vi "fw103_with_subvi_errorhandle.vi"(7 "SerialNumber":string="40154488", 8 "Set position\n(deg) (float)":dbl, 9 "Move (bool)":bool, 10 "Stop all (bool)":bool) -> (0 "Polling reference":refnum<k24>, 1 "Method reference":refnum<k24>, 3 "Current position (deg) (float)":i32)   [LabVIEW 2020]
uses:
  C:/Users/OPMuser/Documents/labview/fw103/Thorlabs.MotionControl.Benchtop.StepperMotorCLI.dll
  Thorlabs.MotionControl.Benchtop.StepperMotorCLI.dll
  <extravilib>/ChannelInstances/Tag-bool.lvlib
  <extravilib>/ChannelInstances/Stream-bool.lvlib
  <vilib>/ErrorRing/Error Ring.xnode
  <vilib>/Utility/error.llb/Error Cluster From Error Code.vi
  C:/Users/OPMuser/Documents/labview/fw103/Thorlabs.MotionControl.Controls.dll
  Thorlabs.MotionControl.Controls.dll
panel:
  in  "Set/Move":dbl
  # "Filter wheel control"
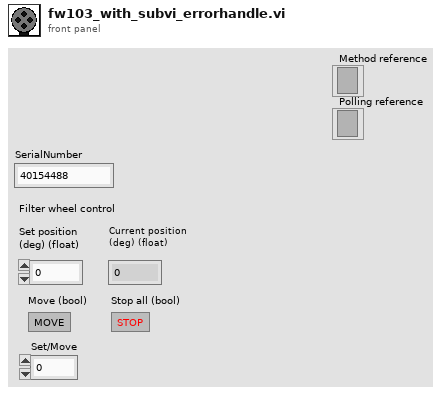
[diagram p1: front panel]
types:
  T1 = typedef "Tag-bool.lvlib/))Channel.ctl" = refnum<queue>
  T2 = typedef "Stream-bool.lvlib/)Channel.ctl" = refnum<queue>
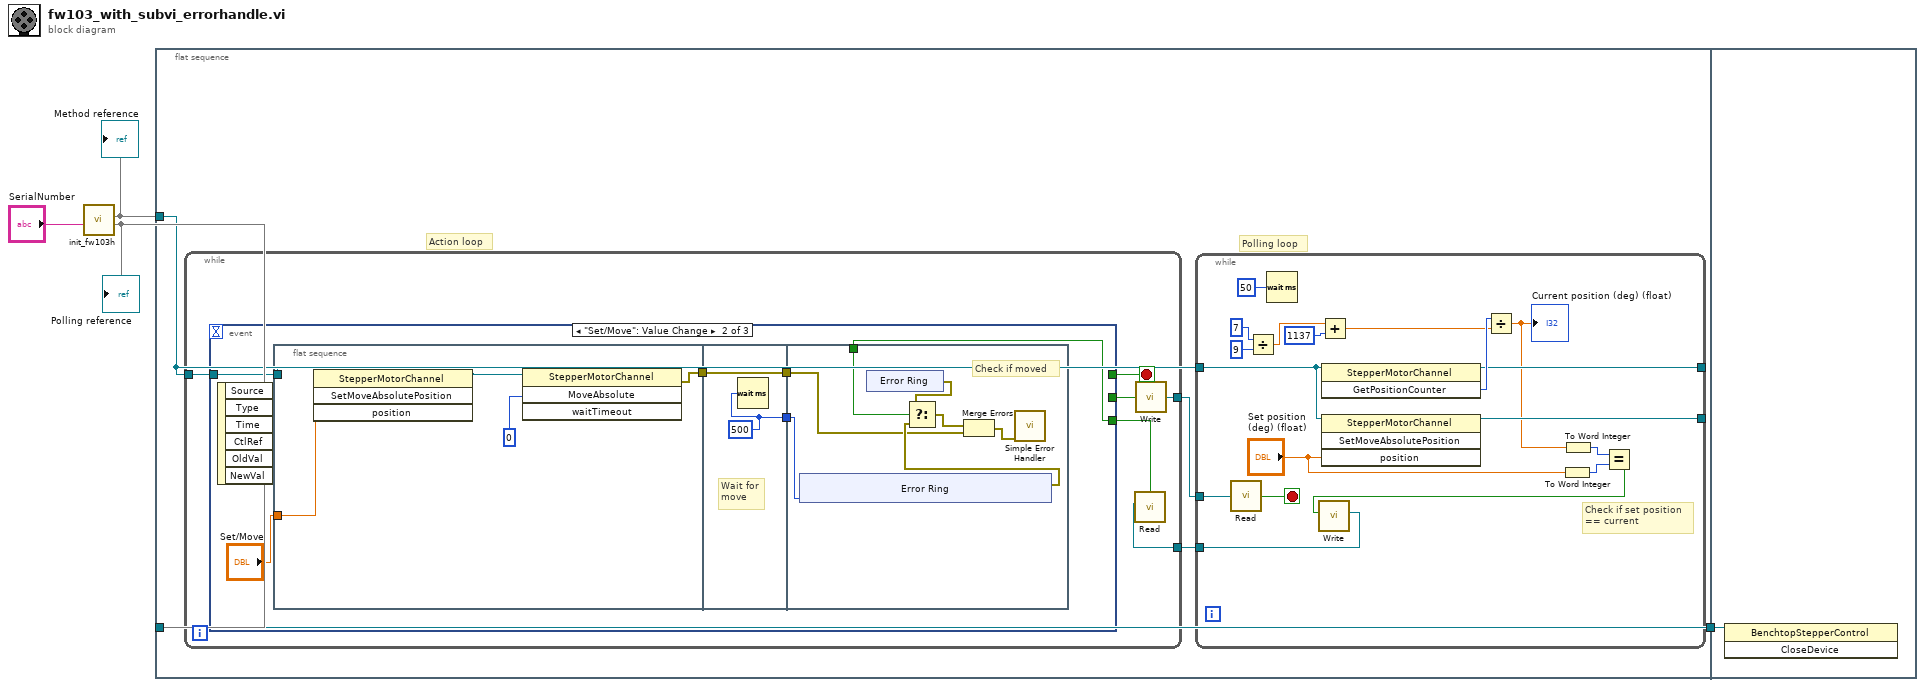
[diagram p0: block diagram]
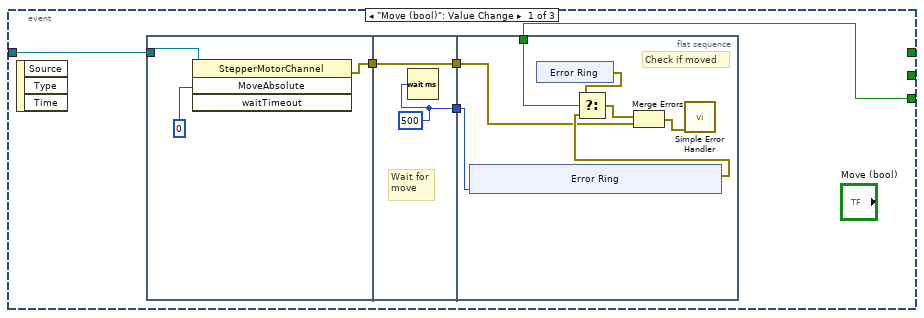
[diagram p2: hidden frame]
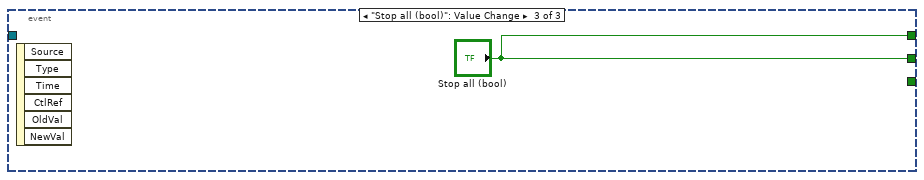
[diagram p3: hidden frame]
diagram:
  n1 = call "init_fw103h.vi"("SerialNumber"="SerialNumber") -> (1:w2, 2:w4)  [unwired: 8 in, 1 out]
  "Method reference" <- w4
  "Polling reference" <- w2
  n2 = flat-sequence {
    tunnel: w4 -> [w6]
    tunnel: [w8] -> w3
    tunnel: w2 -> [w8]
    tunnel: w3 -> [w87]
    frame #0 {
      # "Action loop"
      # "Polling loop"
      n3 = while {
        tunnel: [w12] -> w7
        tunnel: w6 -> [w11]
        tunnel: w5 -> [w9]
        stop <- w14 stop-if-true
        n4 = call <extravilib>:"Read.vi"("channel"=w9) -> ("element"=w10:bool)  [unwired: 6 in, 4 out]
        n5 = event shown="[1] \"Set/Move\": Value Change" {
          selector: _ -> [_ _ _]
          dyn-events: _ -> [_ _ _]
          timeout: _ -> [_ _ _]
          tunnel: [_ _ "Stop all (bool)"] -> w14
          tunnel: [_ _ "Stop all (bool)"] -> w13
          tunnel: w11 -> [w19 w42 _]
          tunnel: w10 -> [w17 w41 _]
          event "Move (bool)": Value Change {
            n6 = event-data() -> ()  [unwired: 1 in, 3 out]
            n7 = flat-sequence {
              tunnel: w19 -> [w21]
              tunnel: [w20] -> w15
              tunnel: [w24] -> w18
              tunnel: [w23] -> w16
              tunnel: w15 -> [w23]
              tunnel: w18 -> [w31]
              tunnel: w17 -> [w30]
              tunnel: w16 -> [w26]
              frame #0 {
                n8 = invoke class="StepperMotorChannel" method="MoveAbsolute"(reference=w21, "waitTimeout"=0) -> (error out=w20:errorcluster)  [unwired: 2 in, 3 out]
              }
              frame #1 {
                w24 = 500 ("waitTimeout")
                # "Wait for\nmove"
                n9 = Wait (ms)(milliseconds to wait=w24) -> ()  [unwired: 1 out]
              }
              frame #2 {
                # "Check if moved"
                n10 = xnode "Error Ring"("parameter 0"=w31) -> ("error out"=w28:errorcluster)
                n11 = xnode "Error Ring"() -> ("error out"=w29:errorcluster)
                n12 = Select(t=w29, s=w30, f=w28) -> (s? t:f=w27:errorcluster)
                n13 = Merge Errors(w27, w26) -> (w25:errorcluster)
                n14 = call <vilib>:"Simple Error Handler.vi"("error in (no error)"=w25) -> ()  [unwired: 4 in, 5 out]
              }
            }
          }
          event "Set/Move": Value Change {
            n15 = event-data() -> ()  [unwired: 1 in, 6 out]
            n16 = flat-sequence {
              tunnel: [w49] -> w45
              tunnel: "Set/Move" -> [w48]
              tunnel: w42 -> [w47]
              tunnel: [w52] -> w44
              tunnel: [w51] -> w43
              tunnel: w45 -> [w51]
              tunnel: w44 -> [w59]
              tunnel: w41 -> [w58]
              tunnel: w43 -> [w54]
              frame #0 {
                n17 = invoke class="StepperMotorChannel" method="SetMoveAbsolutePosition"(reference=w47, "position"=w48) -> (reference out=w46:refnum<k24>)  [unwired: 2 in, 3 out]
                n18 = invoke class="StepperMotorChannel" method="MoveAbsolute"(reference=w46, "waitTimeout"=0) -> (error out=w49:errorcluster)  [unwired: 2 in, 3 out]
              }
              frame #1 {
                w52 = 500 ("waitTimeout")
                # "Wait for\nmove"
                n19 = Wait (ms)(milliseconds to wait=w52) -> ()  [unwired: 1 out]
              }
              frame #2 {
                # "Check if moved"
                n20 = xnode "Error Ring"("parameter 0"=w59) -> ("error out"=w56:errorcluster)
                n21 = xnode "Error Ring"() -> ("error out"=w57:errorcluster)
                n22 = Select(t=w57, s=w58, f=w56) -> (s? t:f=w55:errorcluster)
                n23 = Merge Errors(w55, w54) -> (w53:errorcluster)
                n24 = call <vilib>:"Simple Error Handler.vi"("error in (no error)"=w53) -> ()  [unwired: 4 in, 5 out]
              }
            }
          }
          event "Stop all (bool)": Value Change {
            n25 = event-data() -> ()  [unwired: 1 in, 6 out]
          }
        }
        n26 = call <extravilib>:"Write.vi"("element"=w13) -> ("channel"=w12:T1)  [unwired: 1 out]
      }
      n27 = while {
        tunnel: w6 -> [w78]
        tunnel: [w79] -> _
        tunnel: [w75] -> _
        tunnel: w7 -> [w77]
        tunnel: [w69] -> w5
        stop <- w76 stop-if-true
        # "Check if set position\n== current"
        n28 = call <extravilib>:"Read.vi"("channel"=w77) -> ("element"=w76:bool)  [unwired: 1 in, 1 out]
        n29 = Divide(x=7, y=9) -> (x/y=w82:dbl)
        n30 = Wait (ms)(milliseconds to wait=u32 50) -> ()  [unwired: 1 out]
        n31 = Add(x=w82, y=1137) -> (x+y=w80:dbl)
        n32 = invoke class="StepperMotorChannel" method="GetPositionCounter"(reference=w78) -> (reference out=w79:refnum<k24>, "GetPositionCounter"=w83:i32)  [unwired: 2 in, 1 out]
        n33 = invoke class="StepperMotorChannel" method="SetMoveAbsolutePosition"(reference=w78, "position"="Set position\n(deg) (float)") -> (reference out=w75:refnum<k24>)  [unwired: 2 in, 3 out]
        n34 = Divide(x=w83, y=w80) -> (x/y=w74:dbl)
        "Current position (deg) (float)" <- w74
        n35 = To Word Integer(number="Set position\n(deg) (float)") -> (16bit integer=w71:i16)
        n36 = To Word Integer(number=w74) -> (16bit integer=w72:i16)
        n37 = Equal?(x=w72, y=w71) -> (x = y?=w70:bool)
        n38 = call <extravilib>:"Write.vi"("element"=w70) -> ("channel"=w69:T2)  [unwired: 8 in, 2 out]
      }
    }
    frame #1 {
      n39 = invoke class="BenchtopStepperControl" method="CloseDevice"(reference=w87) -> ()  [unwired: 2 in, 3 out]
    }
  }
